vi "Get Path Regex.vi"(8 "error in (no error)":errorcluster, 11 "TimerStatusController in":refnum<class "TimerStatusController.lvclass">) -> (0 "error out":errorcluster, 2 "Path Regex":string, 3 "TimerStatusController out":refnum<class "TimerStatusController.lvclass">)   [LabVIEW 2020, in "Timer Demo.lvlib" / "TimerStatusController.lvclass"]
uses:
  TimerStatusController.lvclass
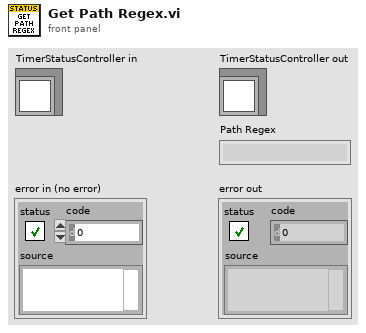
[diagram p1: front panel]
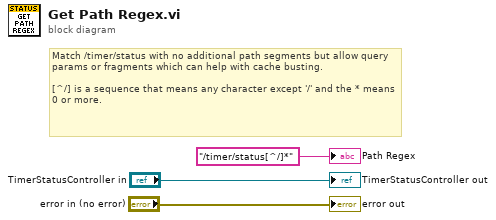
[diagram p0: block diagram]
diagram:
  # "Match /timer/status with no additional path segments but allow query params or fragments which can help with cache busting.\n\n[^/] is a sequence that means any character except '/' and the * means 0 or more."
  "error out" <- "error in (no error)"
  "TimerStatusController out" <- "TimerStatusController in"
  "Path Regex" <- "/timer/status[^/]*" ("Path Regex")
